vi "23384_Davis_Poku_Amankwa_Amankwa.DavisPoku.MNE1201.2.3_348253_1592955325.vi"() -> ()   [LabVIEW 2018]
panel:
  out "Waveform Chart":dbl(graph)
  in  "stop":bool
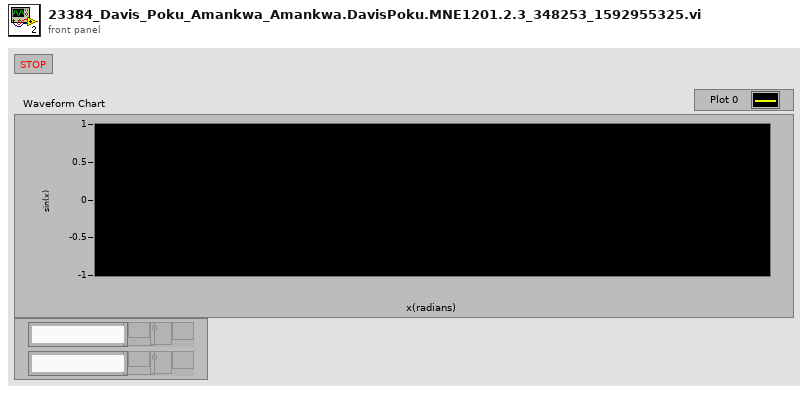
[diagram p1: front panel]
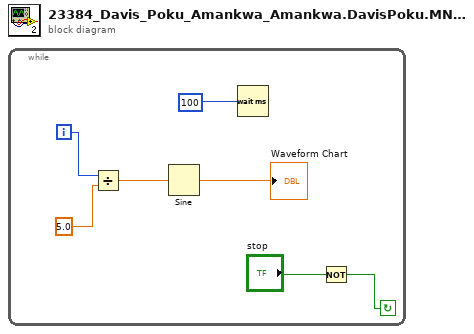
[diagram p0: block diagram]
diagram:
  n1 = while {
    i -> [w5]
    stop <- w6 continue-if-true
    n2 = Divide(x=w5, y=5.0) -> (x/y=w3:dbl)
    n3 = Sine(x=w3) -> (sin(x)=→"Waveform Chart":dbl)
    n4 = Wait (ms)(milliseconds to wait=100) -> ()  [unwired: 1 out]
    n5 = Not(x="stop") -> (.not. x?=w6:bool)
  }
